vi "SPI_Write_Protocol.vi"(8 "rising_edge":bool, 9 "bit_index":i32, 10 "message":bool[](array[boolean])=[FALSE, FALSE, FALSE, FALSE, FALSE, FALSE, FALSE, FALSE, FALSE, FALSE, FALSE, FALSE, FALSE, FALSE, FALSE, FALSE, FALSE, FALSE, FALSE, FALSE, FALSE, FALSE, FALSE, FALSE, FALSE, FALSE, FALSE, FALSE, FALSE, FALSE, FALSE, FALSE], 11 "Register_adress":bool[](array[boolean])=[FALSE, FALSE, FALSE, FALSE, FALSE, FALSE, FALSE, FALSE, FALSE, FALSE, FALSE, FALSE, FALSE, FALSE, FALSE, FALSE, FALSE, FALSE, FALSE, FALSE, FALSE, FALSE, FALSE, FALSE, FALSE, FALSE, FALSE, FALSE, FALSE, FALSE, FALSE, FALSE]) -> ()   [LabVIEW 2019]
doc: "This Vi write a slave message based on SPI protocol. It works with a clock handler and inside a loop"
uses:
  <vilib>/rvi/eio/common/nirviEmuTemplateMethod_errors.vi
  <vilib>/eio/EIONode/EIONode.xnode
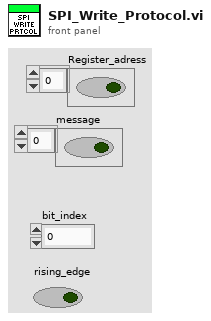
[diagram p1: front panel]
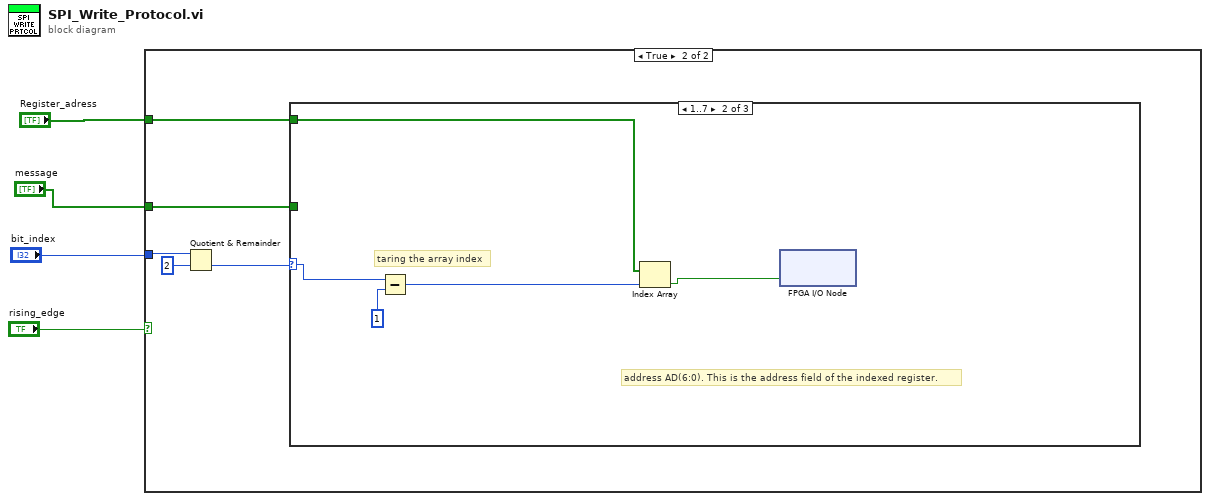
[diagram p0: block diagram]
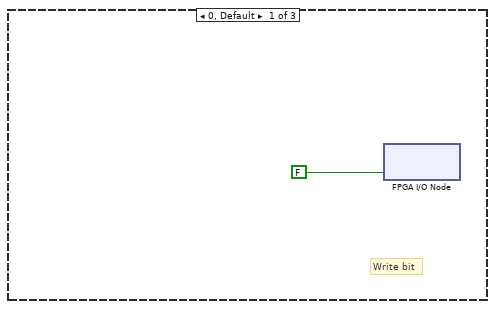
[diagram p3: hidden frame]
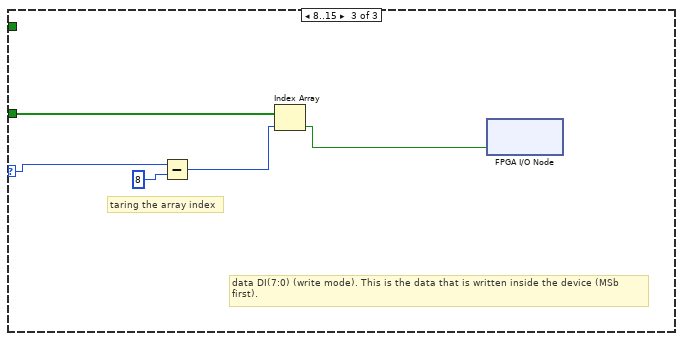
[diagram p4: hidden frame]
diagram:
  n1 = case shown="True" "rising_edge" {
    tunnel: "bit_index" -> [_ w9]
    tunnel: "Register_adress" -> [_ w6]
    tunnel: "message" -> [_ w5]
    frame False {
    }
    frame True {
      n2 = Quotient & Remainder(x=w9, y=2) -> (floor(x/y)=w7:i32)  [unwired: 1 out]
      n3 = case shown="1..7" w7 {
        selector: w7 -> [_ w15 w18]
        tunnel: w6 -> [_ w12 _]
        tunnel: w5 -> [_ _ w20]
        frame 0, Default {
          # "Write bit"
          n4 = xnode "FPGA I/O Node"("SDI"=FALSE) -> ()  [unwired: 1 in, 1 out]
        }
        frame 1..7 {
          # "taring the array index"
          # "address AD(6:0). This is the address field of the indexed register."
          n5 = Subtract(x=w15, y=1) -> (x-y=w13:i32)
          n6 = Index Array(array=w12, index=w13) -> (element=w11:bool)
          n7 = xnode "FPGA I/O Node"("SDI"=w11) -> ()  [unwired: 1 in, 1 out]
        }
        frame 8..15 {
          # "taring the array index"
          # "data DI(7:0) (write mode). This is the data that is written inside the device (MSb\nfirst)."
          n8 = Subtract(x=w18, y=8) -> (x-y=w16:i32)
          n9 = Index Array(array=w20, index=w16) -> (element=w19:bool)
          n10 = xnode "FPGA I/O Node"("SDI"=w19) -> ()  [unwired: 1 in, 1 out]
        }
      }
    }
  }
